vi "InfoOfPlayerCluster2StringArray.vi"(1 "玩家信息":T1) -> (0 "数组":string[](array[string]))   [LabVIEW 2019]
uses:
  ctl/InfoOfPlayer.ctl
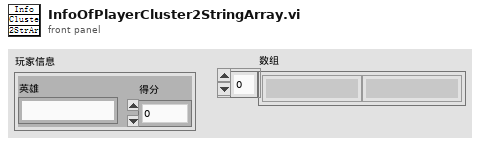
[diagram p1: front panel]
types:
  T1 = typedef "InfoOfPlayer.ctl" = cluster{"得分":i32, "英雄":string}
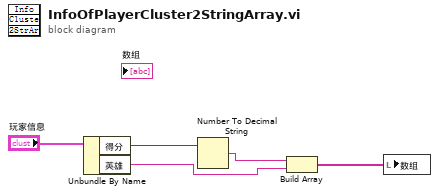
[diagram p0: block diagram]
diagram:
  n1 = Unbundle By Name("玩家信息") -> ("得分"=w4:i32, "英雄"=w2:string)
  n2 = Number To Decimal String(number=w4) -> (decimal integer string=w3:string)  [unwired: 1 in]
  n3 = Build Array(w3, w2) -> (w1:string[])
  n4 = local write "数组"(w1) -> ()
